vi "Configure Cable Guard Mode.vi"(8 "error in (no error)":errorcluster, 10 "Guard Mode  (0: Ohms Guard)":u16(ring) items=["Ohms Guard", "Cable Guard"], 11 "VISA resource name":refnum<visa-resource-name>) -> (0 "error out":errorcluster, 3 "VISA resource name out":refnum<visa-resource-name>)   [LabVIEW 2017, in "Keithley 24XX.lvlib"]
doc: "Configures the cable guard between a low impedance guard and a high impedance guard designed to reduce current leakage."
uses:
  Keithley 24XX.lvlib
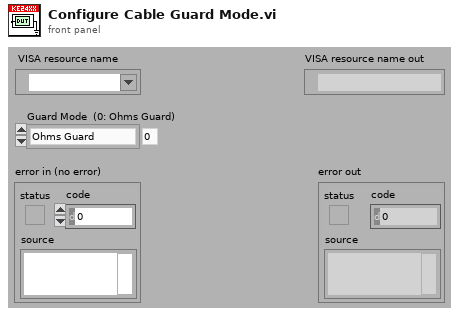
[diagram p1: front panel]
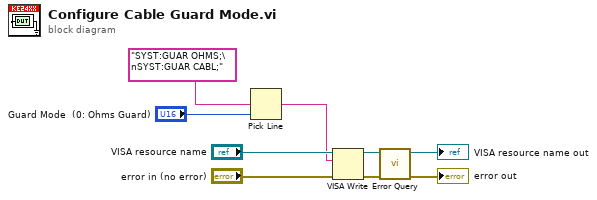
[diagram p0: block diagram]
diagram:
  n1 = Pick Line(multi-line string="SYST:GUAR OHMS;\nSYST:GUAR CABL;", line index="Guard Mode  (0: Ohms Guard)") -> (output string=w1:string)  [unwired: 1 in]
  n2 = VISA Write(VISA resource name="VISA resource name", write buffer=w1, error in (no error)="error in (no error)") -> (VISA resource name out=w5:refnum<visa-resource-name>, error out=w4:errorcluster)  [unwired: 1 out]
  n3 = call "Error Query.vi"("error in (no error)"=w4, "VISA resource name"=w5) -> ("error out"=→"error out":errorcluster, "VISA resource name out"=→"VISA resource name out":refnum<visa-resource-name>)  [unwired: 6 in, 2 out]
